vi "Set NI-SWITCH Reservation Group.vi"(8 "error in":errorcluster, 10 "reservation group":string, 11 "ni-switch custom device in":T1 format="%.0x") -> (0 "error out":errorcluster, 3 "ni-switch custom device out":T1 format="%.0x")   [LabVIEW 2017, in "NI-SWITCH Scripting.lvlib"]
doc: "Sets the reservation group for the SLSC Switch custom device."
uses:
  NI-SWITCH Scripting.lvlib
  <vilib>/NI Veristand/Custom Device API/Custom Device Item Ref.ctl
  SLSC Scripting Constants.vi
  <vilib>/NI Veristand/Custom Device API/Set Item Property (String).vi
  <vilib>/NI VeriStand/Custom Device API/Custom Device API.lvlib
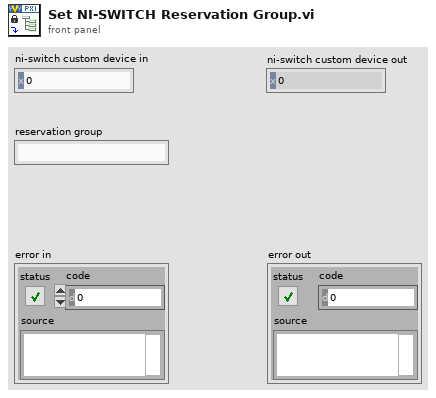
[diagram p1: front panel]
types:
  T1 = typedef "Custom Device API.lvlib/Custom Device Item Ref.ctl" = u64
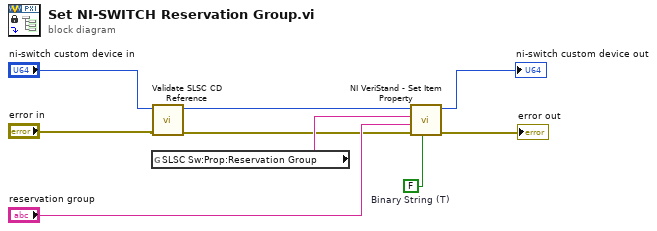
[diagram p0: block diagram]
diagram:
  w6 = FALSE  # Binary String (T)
  n1 = global read "SLSC Scripting Constants.vi" "SLSC Sw:Prop:Reservation Group"() -> (w7:string)
  n2 = call "Validate SLSC CD Reference.vi"("error in"="error in", "ni-switch custom device in"="ni-switch custom device in") -> ("error out"=w3:errorcluster, "ni-switch custom device out"=w1:T1)  [unwired: 8 in]
  n3 = call-poly <vilib>:"NI VeriStand - Set Item Property.vi"("Binary String (T)"=w6, "error in (no error)"=w3, "Value"="reservation group", "Property Name"=w7, "Item Ref in"=w1) -> ("error out"=→"error out":errorcluster, "Item Ref out"=→"ni-switch custom device out":T1)  [unwired: 4 in, 1 out]
